vi "CommunicationTool.vi"(0 "VISA资源名称":refnum<visa-resource-name>="COM1", 1 "SN":string, 2 "ModelNumber":string, 5 "通信协议名称":string, 7 "Slot":T1, 9 "DelayTime":u32=1000, 11 "error in":errorcluster, 12 "Debug":bool) -> (3 "字符串数值":bool=TRUE, 4 "响应":string="ÿÿÿÿÿÿÿÿÿÿÿÿÿÿÿÿÿÿÿÿÿÿÿÿÿÿÿ", 6 "反馈结果":bool, 10 "CMD":string, 14 "data":string, 15 "error out":errorcluster)   [LabVIEW 2013]
doc: "本范例根据用户指示，对串口执行读写操作。范例运行时可按下“写入”或“读取”按钮，以及修改“读数”。\n\n设置的串口参数必须匹配连接仪器或设备的参数。本范例中，“读数”参数可指定串口读取的字节数。如端口字节超过指定的字节数，超出部分将不会被读取。如端口字节数少于指定的字节数，将返回超时错误。\n\n本范例可扩展流控制选项以包括XON和XOFF，从而允许用户选择控制字符。同时，用户可启用或禁用中止符。部分设备需要通过终止符确定命令字符串的结束位置。部分设备将发送终止符以说明待读取数据的末端。本范例演示了缓冲区中检测到终止符时，结束“读取”操作或添加终止符至“写入”数据末端的方法。"
uses:
  SystemCode/SysControl/Slot.ctl
  <vilib>/Utility/NIReport.llb/NI_report.lvclass
  SourceCode/CCID info.ctl
  SourceCode/GlobalValue.vi
  <vilib>/Utility/error.llb/Error Cluster From Error Code.vi
  <vilib>/addons/_office/excel.llb/Excel Get Data ([str]).vi
  <vilib>/Utility/file.llb/Write To Spreadsheet File (string).vi
  <vilib>/Utility/file.llb/Read From Spreadsheet File (string).vi
  <vilib>/ErrorRing/Error Ring.xnode
  <vilib>/addons/_office/NI_ReportGenerationToolkit.lvlib
  <vilib>/Utility/NIReport.llb/Excel/NI_Excel.lvclass
panel:
  out "Time(ms)":u32
  out "SerNO":string
  out "硬件版本":string
  out "终端ID":string
  out "CCID":string="PASS"
  out "生产日期":string
  out "字符串":string
  out "x-y":u32
  out "已删除的部分":u8[](array[numeric]) format="%x"
  out "读取缓冲区":string
  out "数据Hex":string[](array[string])
  out "数据ASCII":string[](array[string])
  out "数据类型":string[](array[string])
  in  "命令列表":u16(ring)=17
  out "Write":bool
  out "Read":bool
  out "ConfigPath":string="C:\\Users\\dell\\Desktop\\ExcelReport.vi"
  out "Data":string
  out "DataType":string
  out "命令":string
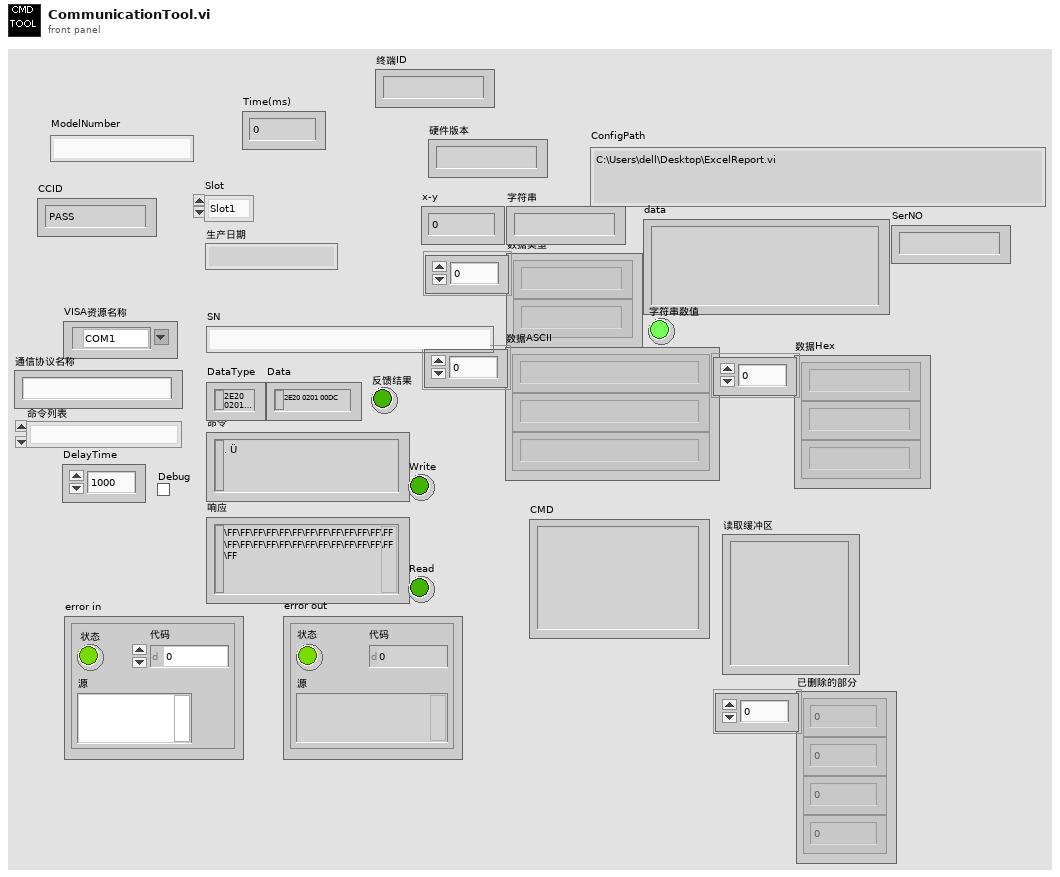
[diagram p1: front panel]
types:
  T1 = typedef "Slot.ctl" = enum16{"Slot1", "Slot2", "Slot3", "Slot4"}
  T2 = enum32{"invalid app kind", "Development System", "Run Time System", "Student Edition", "Embedded LabVIEW", "Evaluation", "Custom"}
  T3 = enum16{"maximized", "minimized", "normal", "no change"}
  T4 = enum16{"Standard Report", "HTML", "Word", "Excel"}
  T5 = typedef "CCID info.ctl" = enum16{"Fw Ver", "HW Ver", "CCID", "WiFiName", "DevID"}
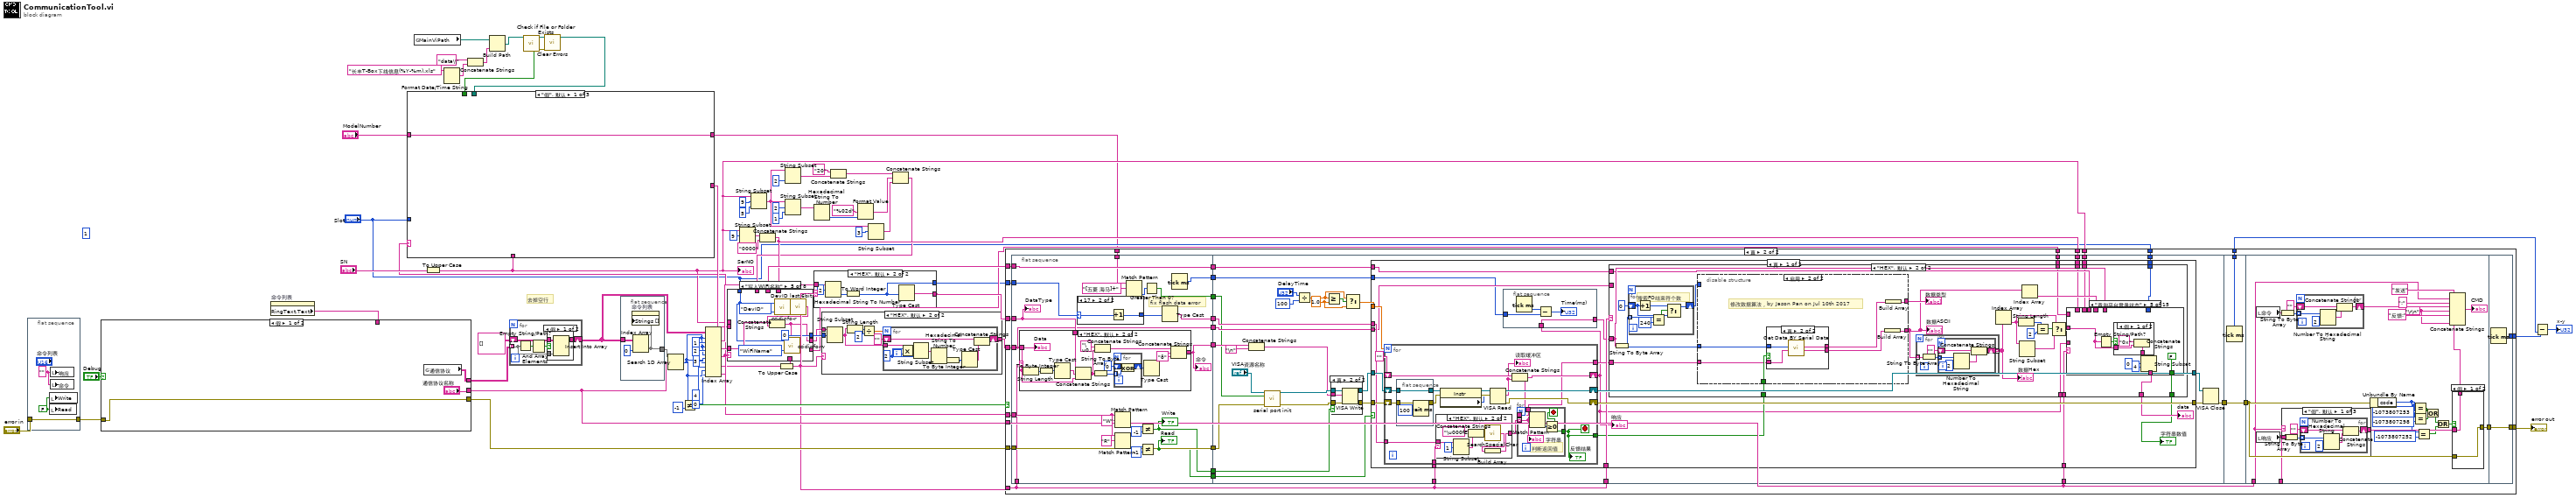
[diagram p0: block diagram]
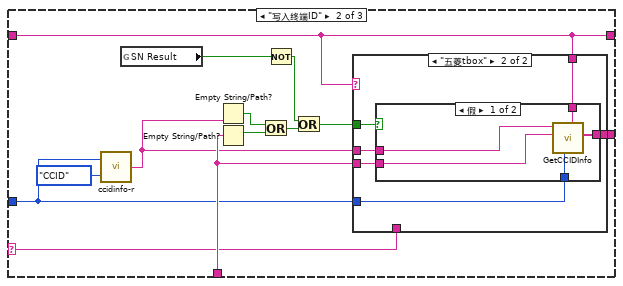
[diagram p2: hidden frame]
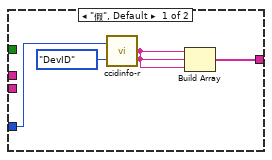
[diagram p3: hidden frame]
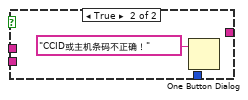
[diagram p4: hidden frame]
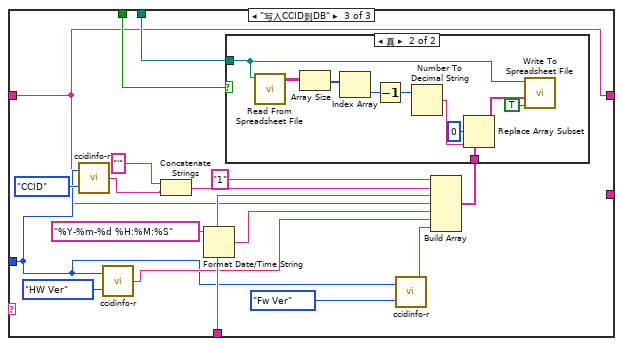
[diagram p5: hidden frame]
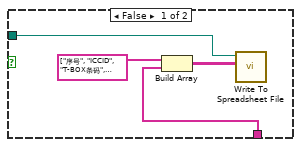
[diagram p6: hidden frame]
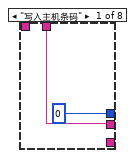
[diagram p7: hidden frame]
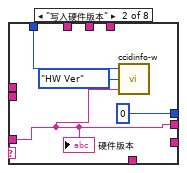
[diagram p8: hidden frame]
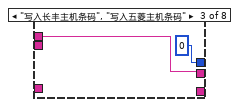
[diagram p9: hidden frame]
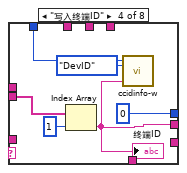
[diagram p10: hidden frame]
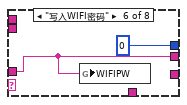
[diagram p11: hidden frame]
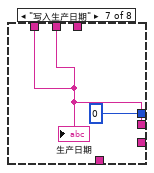
[diagram p12: hidden frame]
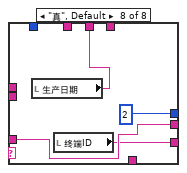
[diagram p13: hidden frame]
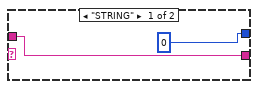
[diagram p14: hidden frame]
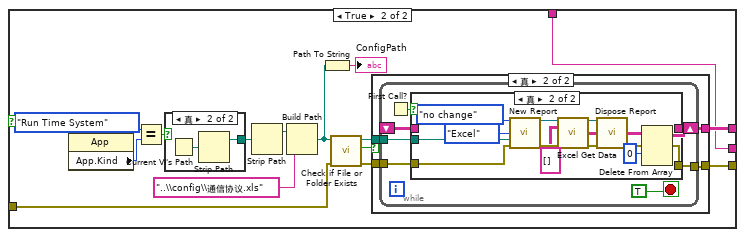
[diagram p17: hidden frame]
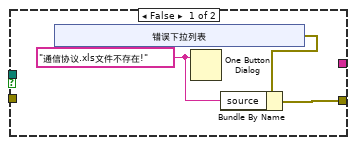
[diagram p18: hidden frame]
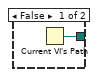
[diagram p20: hidden frame]
diagram:
  (unwired) 1
  # "去掉空行"
  n1 = flat-sequence {
    tunnel: "error in" -> [w71]
    tunnel: [w71] -> w68
    frame #0 {
      w73 = FALSE ("Read")
      w72 = "" ("响应")
      n2 = local write "Write"(w73) -> ()
      n3 = local write "Read"(w73) -> ()
      n4 = local write "响应"(w72) -> ()
      n5 = local write "命令"(w72) -> ()
    }
  }
  n6 = property on="命令列表" class="Ring (严格)"() -> ("RingText.Text"=w67:string)  [unwired: 2 in, 2 out]
  n7 = case shown="假" "Debug" {
    tunnel: [w75 w80] -> w65
    tunnel: w68 -> [w75 w79]
    tunnel: ["通信协议名称" w77] -> w56
    tunnel: [w74 w78] -> w5
    tunnel: w67 -> [_ w77]
    frame False {
      n8 = global read "GlobalValue.vi" "通信协议"() -> (w74:string[][])
    }
    frame True {
      n9 = property class="App"() -> ("App.Kind"=w89:T2)  [unwired: 2 in, 2 out]
      n10 = Equal?(x=T2."Run Time System" ("y"), y=w89) -> (x = y?=w91:bool)
      n11 = case shown="真" w91 {
        tunnel: [w125 w127] -> w90
        frame False {
          n12 = Current VI's Path() -> (path=w125:path)
        }
        frame True {
          n13 = Current VI's Path() -> (path=w126:path)
          n14 = Strip Path(path=w126) -> (stripped path=w127:path)  [unwired: 1 out]
        }
      }
      n15 = Strip Path(path=w90) -> (stripped path=w84:path)  [unwired: 1 out]
      n16 = Build Path(base path=w84, name or relative path="..\\config\\通信协议.xls" ("连接的字符串")) -> (appended path=w86:path)
      n17 = Path To String(path=w86) -> (string=→"ConfigPath":string)
      n18 = call <vilib>:"Check if File or Folder Exists.vi"("error in (no error)"=w79, "path"=w86) -> ("error out"=w81:errorcluster, "file or folder exists?"=w83:bool, "dup path"=w82:path)  [unwired: 7 out]
      n19 = case shown="真" w83 {
        tunnel: w82 -> [_ w102]
        tunnel: w81 -> [_ w101]
        tunnel: [w93 w100] -> w80
        tunnel: [_ w99] -> w78
        frame False {
          w94 = "通信协议.xls文件不存在!" ("消息")
          n20 = xnode "错误下拉列表"() -> ("错误输出"=w92:errorcluster)
          n21 = One Button Dialog(message=w94) -> ()  [unwired: 1 in, 1 out]
          n22 = Bundle By Name(cluster=w92, "source"=w94) -> (w93:errorcluster)
        }
        frame True {
          n23 = while {
            tunnel: w102 -> [w108]
            tunnel: [w107] -> w100
            tunnel: w101 -> [w106]
            shift-right: [w109] -> w99
            shift-left: _ -> [w104]
            stop <- TRUE stop-if-true
            n24 = First Call?() -> (First Call?: T/F=w103:bool)
            n25 = case shown="真" w103 {
              tunnel: [w111 w115] -> w109
              tunnel: w108 -> [_ w114]
              tunnel: [w110 w113] -> w107
              tunnel: w106 -> [w110 w112]
              tunnel: w104 -> [w111 _]
              frame False {
              }
              frame True {
                n26 = call <vilib>:"New Report.vi"("window state (normal)"=T3."no change", "report type"=T4."Excel", "template (empty)"=w114, "error in (no error)"=w112) -> ("report out"=w120:refnum<class "NI_report.lvclass">, "error out"=w121:errorcluster)  [unwired: 2 in, 8 out]
                n27 = call-poly <vilib>:"Excel Get Data.vi"("report in"=w120, "data type"=string[][] [], "error in (no error)"=w121) -> ("report out"=w117:refnum<class "NI_report.lvclass">, "data"=w122:string[][], "error out"=w116:errorcluster)  [unwired: 10 in]
                n28 = call-dynamic "Dispose Report.vi"("report in"=w117, "error in (no error)"=w116) -> ("error out"=w113:errorcluster)  [unwired: 3 in, 10 out]
                n29 = Delete From Array(array=w122, index (row)=0 ("索引 (行)")) -> (array with subset deleted=w115:string[][])  [unwired: 2 in, 1 out]
              }
            }
          }
        }
      }
    }
  }
  n30 = global read "GlobalValue.vi" "MainViPath"() -> (w11:path)
  n31 = To Upper Case(1:"SN") -> (0:w15:string)
  "SerNO" <- w15
  n32 = Format Date/Time String(time format string (%c)="长丰T-Box下线信息(%Y-%m).xls" ("时间格式字符串(%c)")) -> (date/time string=w13:string)  [unwired: 2 in]
  n33 = Concatenate Strings("data\\" ("字符串"), w13) -> (w10:string)
  n34 = Build Path(base path=w11, name or relative path=w10) -> (appended path=w9:path)
  n35 = for {
    tunnel: w5 -> [w128] mode=indexing
    shift-right: [w131] -> w49
    shift-left: string[][] [] -> [w132]
    n36 = Empty String/Path?(string/path=w128) -> (empty?=w130:bool[])
    n37 = And Array Elements(Boolean array=w130) -> (logical AND=w129:bool)
    n38 = case shown="假" w129 {
      tunnel: w132 -> [w135 w136]
      tunnel: [w134 w136] -> w131
      tunnel: w128 -> [w133 _]
      frame False {
        n39 = Insert Into Array(array=w135, new element=w133) -> (w134:string[][])  [unwired: 2 in]
      }
      frame True {
      }
    }
  }
  n40 = call <vilib>:"Check if File or Folder Exists.vi"("path"=w9) -> ("error out"=w8:errorcluster, "file or folder exists?"=w6:bool, "dup path"=w7:path)  [unwired: 8 in]
  n41 = call <vilib>:"Clear Errors.vi"("error in (no error)"=w8) -> ()  [unwired: 6 in, 1 out]
  n42 = flat-sequence {
    tunnel: [w138] -> w55
    tunnel: w49 -> [w137]
    frame #0 {
      n43 = Index Array(array=w137, index (col)=0 ("禁用的索引 (列)")) -> (element=w138:string[])  [unwired: 1 in]
      n44 = property on="命令列表" class="Ring (严格)"("Strings []"=w138) -> ()  [unwired: 2 in, 2 out]
    }
  }
  n45 = Search 1D Array(1D array=w55, element=w56) -> (index of element=w46:i32)  [unwired: 1 in]
  n46 = Not Equal?(x=w46, y=-1) -> (x != y?=w60:bool)
  n47 = Index Array(array=w49, index (row) #1=w46, index (col) #1=1 ("索引 (列)"), index (row) #2=w46, index (col) #2=2 ("索引 (列)"), index (row) #3=w46, index (col) #3=3 ("索引 (列)"), index (row) #4=w46, index (col) #4=4 ("禁用的索引 (列)"), index (row) #5=w46, index (col) #5=0 ("禁用的索引 (列)")) -> (element #1=w59:string, element #2=w44:string, element #3=w51:string, element #4=w53:string, element #5=w17:string)
  n48 = case shown="\"假\", 默认" w17 {
    selector: w17 -> [_ w142 _]
    tunnel: [_ w153 _] -> w20
    tunnel: "ModelNumber" -> [w140 w141 w170]
    tunnel: w15 -> [_ w146 w185]
    tunnel: w7 -> [_ _ w181]
    tunnel: w6 -> [_ _ w180]
    tunnel: "Slot" -> [_ w145 w172]
    tunnel: [w140 w141 w170] -> w2
    frame "假", Default {
    }
    frame "写入终端ID" {
      n49 = call "ccidinfo-r.vi"("Data Type"=CCID_info."CCID", "Slot"=w145) -> ("Data"=w143:string)
      n50 = global read "GlobalValue.vi" "SN Result"() -> (w152:bool)
      n51 = Empty String/Path?(string/path=w143) -> (empty?=w151:bool)
      n52 = Empty String/Path?(string/path=w146) -> (empty?=w150:bool)
      n53 = Or(x=w151, y=w150) -> (x .or. y?=w148:bool)
      n54 = Not(x=w152) -> (.not. x?=w149:bool)
      n55 = Or(x=w149, y=w148) -> (x .or. y?=w147:bool)
      n56 = case shown="\"五菱tbox\"" w141 {
        tunnel: [w157 w163] -> w153
        tunnel: w147 -> [_ w162]
        tunnel: w141 -> [_ w161]
        tunnel: w146 -> [_ w160]
        tunnel: w145 -> [w155 w159]
        tunnel: w143 -> [_ w158]
        tunnel: w142 -> [_ _]
        frame "假", Default {
          n57 = call "ccidinfo-r.vi"("Data Type"=CCID_info."DevID", "Slot"=w155) -> ("Data"=w154:string)
          n58 = Build Array(w154, w154, w154) -> (w157:string[])
        }
        frame "五菱tbox" {
          n59 = case shown="假" w162 {
            tunnel: [w168 _] -> w163
            tunnel: w158 -> [w167 _]
            tunnel: w160 -> [w166 _]
            tunnel: w161 -> [w165 _]
            tunnel: w159 -> [w164 _]
            frame False {
              n60 = call "GetCCIDInfo.vi"("table name"=w165, "Slot"=w164, "SerNO"=w166, "CCID"=w167) -> ("CCID信息"=w168:string[])  [unwired: 7 in]
            }
            frame True {
              n61 = One Button Dialog(message="CCID或主机条码不正确！" ("消息")) -> ()  [unwired: 1 in, 1 out]
            }
          }
        }
      }
    }
    frame "写入CCID到DB" {
      n62 = call "ccidinfo-r.vi"("Data Type"=CCID_info."CCID", "Slot"=w172) -> ("Data"=w176:string)
      n63 = call "ccidinfo-r.vi"("Data Type"=CCID_info."HW Ver", "Slot"=w172) -> ("Data"=w174:string)
      n64 = Concatenate Strings("'", w176) -> (w178:string)
      n65 = Format Date/Time String(time format string (%c)="%Y-%m-%d %H:%M:%S" ("时间格式字符串(%c)")) -> (date/time string=w183:string)  [unwired: 2 in]
      n66 = call "ccidinfo-r.vi"("Data Type"=CCID_info."Fw Ver", "Slot"=w172) -> ("Data"=w171:string)
      n67 = Build Array("1", w178, w185, w170, w183, w174, w171) -> (w182:string[])
      n68 = case shown="真" w180 {
        tunnel: w181 -> [w190 w191]
        tunnel: w182 -> [w189 w195]
        frame False {
          n69 = Build Array(string[] ["序号", "ICCID", "T-BOX条码", "设备型号", "生产日期", "硬件版本", "软件版本"], w189) -> (w188:string[][])
          n70 = call-poly <vilib>:"Write To Spreadsheet File.vi"("2D data"=w188, "file path (dialog if empty)"=w190) -> ()  [unwired: 6 in, 1 out]
        }
        frame True {
          n71 = call-poly <vilib>:"Read From Spreadsheet File.vi"("file path (dialog if empty)"=w191) -> ("all rows"=w200:string[][])  [unwired: 6 in, 4 out]
          n72 = Array Size(array=w200) -> (size(s)=w199:i32[])
          n73 = Index Array(array=w199) -> (element=w198:i32)  [unwired: 1 in]
          n74 = Decrement(x=w198) -> (x-1=w197:i32)
          n75 = Number To Decimal String(number=w197) -> (decimal integer string=w193:string)  [unwired: 1 in]
          n76 = Replace Array Subset(array=w195, new element=w193, index=0 ("索引")) -> (w192:string[])
          n77 = call-poly <vilib>:"Write To Spreadsheet File.vi"("append to file? (new file:F)"=TRUE, "1D data"=w192, "file path (dialog if empty)"=w191) -> ()  [unwired: 5 in, 1 out]
        }
      }
    }
  }
  n78 = String Subset(string=w15, offset (0)=9 ("偏移量(0)")) -> (substring=w39:string)  [unwired: 1 in]
  n79 = String Subset(string=w15, offset (0)=9 ("偏移量(0)"), length (rest)=5 ("长度（剩余）")) -> (substring=w27:string)
  n80 = Concatenate Strings(w39, "0000" ("字符串")) -> (w37:string)
  n81 = To Upper Case(1:w51) -> (0:w3:string)
  n82 = String Subset(string=w27, length (rest)=2 ("长度（剩余）")) -> (substring=w34:string)  [unwired: 1 in]
  n83 = String Subset(string=w27, offset (0)=2 ("偏移量(0)"), length (rest)=1 ("长度（剩余）")) -> (substring=w29:string)
  n84 = Hexadecimal String To Number(string=w29) -> (number=w24:u32)  [unwired: 2 in, 1 out]
  n85 = case shown="\"HEX\", 默认" w3 {
    tunnel: w59 -> [w202 w205]
    tunnel: [w202 w204] -> w58
    tunnel: [i16 0 w203] -> w1
    frame "STRING" {
    }
    frame "HEX", Default {
      n86 = Hexadecimal String To Number(string=w205, offset=2 ("偏移量")) -> (number=w207:u32)  [unwired: 1 in, 1 out]
      n87 = To Word Integer(number=w207) -> (16bit integer=w203:i16)
      n88 = Type Cast(x=w203) -> (*(type *) &x=w204:string)  [unwired: 1 in]
    }
  }
  n89 = Concatenate Strings("20" ("字符串"), w34) -> (w26:string)
  n90 = Format Value(format string="%02d" ("格式字符串"), value (0)=w24) -> (output string=w22:string)  [unwired: 1 in]
  n91 = String Subset(string=w27, offset (0)=3 ("偏移量(0)")) -> (substring=w25:string)  [unwired: 1 in]
  n92 = Concatenate Strings(w26, w22, w25) -> (w21:string)
  n93 = case shown="\"写入WIFI名称\"" w17 {
    tunnel: w44 -> [_ w210 _ _ w228 w230 _ w237]
    tunnel: [w208 w210 w214 w216 w224 w230 w232 w237] -> w19
    tunnel: [0 ("偏移量(0)") 0 ("偏移量(0)") 0 ("偏移量(0)") 0 ("偏移量(0)") 0 ("偏移量(0)") 0 ("偏移量(0)") 0 ("偏移量(0)") 2 ("偏移量(0)")] -> w43
    tunnel: [_ _ _ _ _ _ w232 w235] -> w41
    tunnel: w37 -> [w208 _ _ _ _ _ _ _]
    tunnel: w21 -> [_ _ _ _ _ _ w232 _]
    tunnel: w15 -> [_ _ w214 _ _ _ _ _]
    tunnel: w20 -> [_ _ _ w220 _ _ _ _]
    tunnel: [_ _ _ _ _ _ _ w234] -> w18
    tunnel: "Slot" -> [_ w212 _ w217 w225 _ _ _]
    tunnel: w3 -> [_ _ _ _ _ _ _ _]
    frame "写入主机条码" {
    }
    frame "写入硬件版本" {
      n94 = call "ccidinfo-w.vi"("Data"=w210, "Data Type"=CCID_info."HW Ver", "Slot"=w212) -> ()  [unwired: 1 in]
      "硬件版本" <- w210
    }
    frame "写入长丰主机条码", "写入五菱主机条码" {
    }
    frame "写入终端ID" {
      n95 = Index Array(array=w220, index=1 ("索引")) -> (element=w216:string)
      "终端ID" <- w216
      n96 = call "ccidinfo-w.vi"("Data"=w216, "Data Type"=CCID_info."DevID", "Slot"=w217) -> ()  [unwired: 1 in]
    }
    frame "写入WIFI名称" {
      n97 = call "ccidinfo-r.vi"("Data Type"=CCID_info."DevID", "Slot"=w225) -> ("Data"=w223:string)
      n98 = call "DevID last 6bit.vi"("Devid"=w223) -> ("结果字符串"=w222:string)  [unwired: 4 in]
      n99 = Concatenate Strings(w228, w222) -> (w224:string)
      n100 = call "ccidinfo-w.vi"("Data"=w224, "Data Type"=CCID_info."WiFiName", "Slot"=w225) -> ()  [unwired: 1 in]
    }
    frame "写入WIFI密码" {
      n101 = global write "GlobalValue.vi" "WIFIPW"(w230) -> ()
    }
    frame "写入生产日期" {
      "生产日期" <- w232
    }
    frame "真", Default {
      n102 = local read "生产日期"() -> (w235:string)
      n103 = local read "终端ID"() -> (w234:string)
    }
  }
  n104 = case shown="\"HEX\", 默认" w3 {
    tunnel: [w238 w243] -> w57
    tunnel: w19 -> [w238 w242]
    tunnel: w43 -> [_ w239]
    frame "ASCII" {
    }
    frame "HEX", Default {
      n105 = String Subset(string=w242, offset (0)=w239) -> (substring=w241:string)  [unwired: 1 in]
      n106 = String Length(string=w241) -> (length=w245:i32)
      n107 = Divide(x=w245, y=2) -> (x/y=w240:dbl)
      n108 = for {
        N: w240 -> [_]
        tunnel: w241 -> [w251]
        shift-right: [w253] -> w243
        shift-left: "" -> [w252]
        i -> [w249]
        w247 = 2 ("x")
        n109 = Multiply(x=w247, y=w249) -> (x*y=w248:i32)
        n110 = String Subset(string=w251, offset (0)=w248, length (rest)=w247) -> (substring=w250:string)
        n111 = Hexadecimal String To Number(string=w250) -> (number=w256:u32)  [unwired: 2 in, 1 out]
        n112 = To Byte Integer(number=w256) -> (8bit integer=w255:i8)
        n113 = Type Cast(x=w255) -> (*(type *) &x=w254:string)  [unwired: 1 in]
        n114 = Concatenate Strings(w252, w254) -> (w253:string)
      }
    }
  }
  n115 = case shown="真" w60 {
    tunnel: w56 -> [w261 w278]
    tunnel: w58 -> [_ w289]
    tunnel: w57 -> [_ w288]
    tunnel: w65 -> [_ w287]
    tunnel: [w257 w285] -> w70
    tunnel: w53 -> [_ w284]
    tunnel: w3 -> [_ w279]
    tunnel: [_ w274] -> w66
    tunnel: [_ w273] -> w48
    tunnel: w41 -> [_ w272]
    tunnel: w37 -> [_ w270]
    tunnel: w15 -> [_ w269]
    tunnel: w18 -> [_ w268]
    tunnel: "Slot" -> [_ w265]
    tunnel: w2 -> [_ w264]
    tunnel: w1 -> [_ w262]
    frame False {
      (unwired) "FF" ("响应")
      n116 = Concatenate Strings(w261, "名称不存在" ("消息")) -> (w258:string)
      n117 = One Button Dialog(message=w258) -> ()  [unwired: 1 in, 1 out]
      n118 = Bundle By Name(cluster=errorcluster {"status"=TRUE, "code"=5000, "source"=""} ("error in 1 (no error)"), "source"=w258) -> (w257:errorcluster)
    }
    frame True {
      n119 = flat-sequence {
        tunnel: w289 -> [w301]
        tunnel: w288 -> [w298]
        tunnel: w287 -> [w312]
        tunnel: [w312] -> w286
        tunnel: w284 -> [w311]
        tunnel: [w304] -> w283
        tunnel: [w303] -> w282
        tunnel: [w302] -> w281
        tunnel: [w290] -> w280
        tunnel: w279 -> [w300]
        tunnel: w272 -> [w299]
        tunnel: [w299] -> w271
        tunnel: [w298] -> w267
        tunnel: [w297] -> w266
        tunnel: w264 -> [w296]
        tunnel: [w293] -> w263
        tunnel: w262 -> [w292]
        tunnel: w286 -> [w365]
        tunnel: w283 -> [w360]
        tunnel: w282 -> [w363]
        tunnel: [w364] -> w277
        tunnel: w281 -> [w339]
        tunnel: w280 -> [w359]
        tunnel: w279 -> [w350]
        tunnel: w279 -> [w349]
        tunnel: w278 -> [w348]
        tunnel: w271 -> [w347]
        tunnel: w270 -> [w346]
        tunnel: w269 -> [w345]
        tunnel: w268 -> [w344]
        tunnel: w267 -> [w343]
        tunnel: w266 -> [w342]
        tunnel: w265 -> [w341]
        tunnel: w263 -> [w336]
        tunnel: w277 -> [w714]
        tunnel: [w714] -> w276
        tunnel: [w713] -> w273
        tunnel: w276 -> [w727]
        tunnel: w278 -> [w715]
        tunnel: [w716] -> _
        tunnel: [w728] -> w275
        tunnel: [w760] -> w285
        tunnel: w275 -> [w760]
        tunnel: [w759] -> w274
        frame #0 {
          # "fix flash data error"
          n120 = case shown="\"HEX\", 默认" w300 {
            tunnel: w298 -> [w317 w329]
            tunnel: [w316 w323] -> w302
            tunnel: w301 -> [w318 w322]
            frame "STRING" {
              n121 = Concatenate Strings(w318, w317) -> (w316:string)
            }
            frame "HEX", Default {
              n122 = String Length(string=w329) -> (length=w320:i32)
              n123 = To Byte Integer(number=w320) -> (8bit integer=w321:i8)
              n124 = Type Cast(x=w321) -> (*(type *) &x=w319:string)  [unwired: 1 in]
              n125 = Concatenate Strings(w322, w319, w329) -> (w332:string)
              n126 = String To Byte Array(string=w332) -> (unsigned byte array=w328:u8[])
              n127 = Concatenate Strings("\u000f" ("HeadCode"), w332) -> (w325:string)
              n128 = for {
                tunnel: w328 -> [w335] mode=indexing
                shift-right: [w333] -> w326
                shift-left: u8 0 ("y") -> [w334]
                n129 = Exclusive Or(1:w335, 2:w334) -> (0:w333:u8)
              }
              n130 = Type Cast(x=w326) -> (*(type *) &x=w330:string)  [unwired: 1 in]
              n131 = Concatenate Strings(w325, w330, "ð" ("字符串")) -> (w323:string)
              "Data" <- w329
            }
          }
          "命令" <- w302
          n132 = case shown="17" w292 {
            selector: w292 -> [w313 w315]
            tunnel: [w313 w314] -> w291
            frame 0, Default {
            }
            frame 17 {
              n133 = Increment(x=w315) -> (x+1=w314:i16)
            }
          }
          n134 = Match Pattern(string=w311, regular expression="W" ("正则表达式")) -> (offset past match=w305:i32)  [unwired: 1 in, 3 out]
          n135 = Match Pattern(string=w311, regular expression="R" ("正则表达式")) -> (offset past match=w306:i32)  [unwired: 1 in, 3 out]
          n136 = Match Pattern(string=w296, regular expression="[五菱 海马]+" ("正则表达式")) -> (offset past match=w294:i32)  [unwired: 1 in, 3 out]
          n137 = Not Equal?(x=w305, y=-1) -> (x != y?=w304:bool)
          "Write" <- w304
          n138 = Not Equal?(x=w306, y=-1) -> (x != y?=w303:bool)
          "Read" <- w303
          n139 = Greater Than 0?(x=w294) -> (x > 0?=w293:bool)
          n140 = Type Cast(x=w291) -> (*(type *) &x=w290:string)  [unwired: 1 in]
          n141 = Tick Count (ms)() -> (millisecond timer value=w297:u32)
          "DataType" <- w301
        }
        frame #1 {
          w356 = 1.0 ("y")
          n142 = Concatenate Strings(w339, "\n") -> (w337:string)
          n143 = call "serial port init.vi"("错误输入（无错误）"=w365, "海马(1)"=w336, "VISA引用句柄输入"="VISA资源名称") -> ("错误输出"=w361:errorcluster, "VISA引用句柄输出"=w362:refnum<visa-resource-name>)  [unwired: 7 in]
          n144 = Divide(x="DelayTime", y=u32 100) -> (x/y=w355:dbl)
          n145 = Greater Or Equal?(x=w355, y=w356) -> (x >= y?=w354:bool)
          n146 = case shown="真" w360 {
            tunnel: w362 -> [w369 w374]
            tunnel: [w369 w373] -> w358
            tunnel: [w368 w372] -> w357
            tunnel: w361 -> [w368 w371]
            tunnel: w337 -> [_ w370]
            frame False {
            }
            frame True {
              n147 = VISA Write(VISA resource name=w374, write buffer=w370, error in (no error)=w371) -> (VISA resource name out=w373:refnum<visa-resource-name>, error out=w372:errorcluster)  [unwired: 1 out]
            }
          }
          n148 = Select(t=w355, s=w354, f=w356) -> (s? t:f=w351:dbl)
          n149 = case shown="真" w363 {
            tunnel: [w396 w712] -> w366
            tunnel: w358 -> [w395 w712]
            tunnel: [w397 w711] -> w367
            tunnel: w357 -> [w394 w711]
            tunnel: w359 -> [w392 _]
            tunnel: w351 -> [w391 _]
            tunnel: w350 -> [w390 _]
            tunnel: w349 -> [w389 _]
            tunnel: w348 -> [w387 _]
            tunnel: w347 -> [w384 _]
            tunnel: w346 -> [w383 _]
            tunnel: w345 -> [w382 _]
            tunnel: w344 -> [w381 _]
            tunnel: w343 -> [w380 _]
            tunnel: w342 -> [w379 _]
            tunnel: w341 -> [w377 _]
            frame True {
              n150 = for {
                N: w391 -> [_]
                shift-right: [w695] -> w397
                shift-left: w394 -> [w685]
                shift-right: [w683] -> w375
                shift-left: "" ("read buffer") -> [w690]
                shift-right: [w694] -> w396
                shift-left: w395 -> [w684]
                tunnel: w392 -> [w680]
                tunnel: w390 -> [w682]
                tunnel: [w681] -> w388
                tunnel: [w679] -> w376
                stop <- w681 stop-if-true
                n151 = flat-sequence {
                  tunnel: w685 -> [w710]
                  tunnel: [w710] -> w686
                  tunnel: [w709] -> w687
                  tunnel: w684 -> [w709]
                  frame #0 {
                    n152 = Wait (ms)(milliseconds to wait=u32 100 ("等待时间（毫秒）")) -> ()  [unwired: 1 out]
                  }
                }
                n153 = case shown="\"HEX\", 默认" w682 {
                  tunnel: [string[] ["0x0000000", "create auto test task"] w701] -> w689
                  tunnel: w680 -> [_ w707]
                  frame "STRING" {
                  }
                  frame "HEX", Default {
                    n154 = String Subset(string=w707, offset (0)=1 ("偏移量(0)")) -> (substring=w704:string)  [unwired: 1 in]
                    n155 = Concatenate Strings("\u000f€" ("正则表达式"), w704) -> (w703:string)
                    n156 = call "SearchSpecialChar.vi"("正则表达式"=w703) -> ("字符串"=w702:string)
                    n157 = Build Array(w702) -> (w701:string[])
                  }
                }
                n158 = property class="Instr"(reference=w687, error in=w686) -> (reference out=w693:refnum<visa-resource-name>, error out=w692:errorcluster, "Serial Settings:Number of Bytes at Serial Port"=w691:u32)
                n159 = VISA Read(VISA resource name=w693, byte count=w691, error in (no error)=w692) -> (VISA resource name out=w694:refnum<visa-resource-name>, read buffer=w688:string, error out=w695:errorcluster)  [unwired: 1 out]
                "读取缓冲区" <- w688
                n160 = Concatenate Strings(w690, w688) -> (w683:string)
                n161 = for {
                  tunnel: w689 -> [w696] mode=indexing
                  tunnel: w683 -> [w698]
                  tunnel: [w697] -> w681
                  tunnel: [w696] -> w679
                  stop <- w697 stop-if-true
                  # "判断返回值"
                  n162 = Match Pattern(string=w698, regular expression=w696) -> (offset past match=w699:i32)  [unwired: 1 in, 3 out]
                  n163 = Greater Or Equal To 0?(x=w699) -> (x >= 0?=w697:bool)
                  "字符串" <- w696
                }
                "反馈结果" <- w681
              }
              "响应" <- w375
              n164 = flat-sequence {
                tunnel: w379 -> [w399]
                tunnel: w375 -> [w398]
                tunnel: [w398] -> w378
                frame #0 {
                  n165 = Tick Count (ms)() -> (millisecond timer value=w400:u32)
                  n166 = Subtract(x=w400, y=w399) -> (x-y=→"Time(ms)":u32)
                }
              }
              n167 = case shown="\"HEX\", 默认" w389 {
                tunnel: w378 -> [w408 w479]
                tunnel: w388 -> [w405 w471]
                tunnel: w387 -> [w409 w487]
                tunnel: [w407 w486] -> w386
                tunnel: [w406 w485] -> w385
                tunnel: w384 -> [_ w476]
                tunnel: w383 -> [_ w475]
                tunnel: w382 -> [w403 w474]
                tunnel: w381 -> [_ w473]
                tunnel: w380 -> [w404 _]
                tunnel: w377 -> [w402 w472]
                tunnel: w376 -> [_ w470]
                tunnel: w375 -> [_ w469]
                frame "STRING" {
                  n168 = case shown="\"查询版本(1701)\"" w409 {
                    tunnel: [w410 w419 w442] -> w407
                    tunnel: [FALSE FALSE FALSE] -> w406
                    tunnel: w408 -> [_ w426 w450]
                    tunnel: w405 -> [w411 _ _]
                    tunnel: w404 -> [_ w421 w444]
                    tunnel: w403 -> [_ _ _]
                    tunnel: w402 -> [_ w417 w440]
                    frame "真", Default {
                      n169 = Select(t="OK", s=w411, f="") -> (s? t:f=w410:string)
                    }
                    frame "查询版本", "查询版本(长丰)" {
                      # "查询版本指令--修改兼容海马,五菱,长丰  --- by Jason Pan on Jan 20th 2017"
                      n170 = Concatenate Strings(w421, "\n" ("字符串")) -> (w420:string)
                      n171 = Match Pattern(string=w426, regular expression=w420) -> (after substring=w425:string)  [unwired: 1 in, 3 out]
                      n172 = for {
                        tunnel: w425 -> [w439]
                        tunnel: [w438] -> w423
                        tunnel: string[] ["\r\n\t1, 0x00000001\r\ncmd>", "\r\n\t0, 0x00000000\r\ncmd>", "\n\t0, 0x00000000", "\r\ncmd>"] -> [w435] mode=indexing
                        tunnel: [w434] -> w424
                        i -> [w434]
                        stop <- w436 stop-if-true
                        n173 = Match Pattern(string=w439, regular expression=w435) -> (before substring=w438:string, offset past match=w437:i32)  [unwired: 1 in, 2 out]
                        n174 = Greater Or Equal To 0?(x=w437) -> (x >= 0?=w436:bool)
                      }
                      n175 = case shown="0, 默认" w424 {
                        tunnel: [w428 w429] -> w422
                        tunnel: w423 -> [w428 w433]
                        frame 0, Default {
                          # "海马/长丰tbox"
                        }
                        frame 3 {
                          # "五菱tbox"
                          n176 = Match Pattern(string=w433, regular expression="app start,version:" ("正则表达式")) -> (after substring=w431:string)  [unwired: 1 in, 3 out]
                          n177 = Match Pattern(string=w431, regular expression="\r\n" ("正则表达式")) -> (before substring=w429:string)  [unwired: 1 in, 3 out]
                        }
                      }
                      n178 = call <vilib>:"Trim Whitespace.vi"("string"=w422) -> ("trimmed string"=w419:string)  [unwired: 1 in]
                      n179 = call "ccidinfo-w.vi"("Data"=w419, "Data Type"=CCID_info."Fw Ver", "Slot"=w417) -> ()  [unwired: 1 in]
                    }
                    frame "查询版本(1701)" {
                      # "查询版本指令--修改兼容海马,五菱,长丰  --- by Jason Pan on Jan 20th 2017"
                      n180 = Concatenate Strings(w444) -> (w443:string)
                      n181 = Match Pattern(string=w450, regular expression=w443) -> (after substring=w449:string)  [unwired: 1 in, 3 out]
                      n182 = for {
                        tunnel: w449 -> [w468]
                        tunnel: [w467] -> w446
                        tunnel: string[] ["\r\nAES", "\nAES"] -> [w464] mode=indexing
                        tunnel: [w463] -> w447
                        i -> [w463]
                        stop <- w465 stop-if-true
                        n183 = Match Pattern(string=w468, regular expression=w464) -> (before substring=w467:string, offset past match=w466:i32)  [unwired: 1 in, 2 out]
                        n184 = Greater Or Equal To 0?(x=w466) -> (x >= 0?=w465:bool)
                      }
                      n185 = case shown="0" w447 {
                        tunnel: [w452 w453 w458] -> w445
                        tunnel: w446 -> [w452 w457 w462]
                        frame -1, Default {
                          # "海马/长丰tbox"
                        }
                        frame 0 {
                          # "tbox/1701"
                          n186 = Match Pattern(string=w457, regular expression="app start,version:" ("正则表达式")) -> (after substring=w455:string)  [unwired: 1 in, 3 out]
                          n187 = Match Pattern(string=w455, regular expression="\r\n" ("正则表达式")) -> (before substring=w453:string)  [unwired: 1 in, 3 out]
                        }
                        frame 1 {
                          # "1701"
                          n188 = Match Pattern(string=w462, regular expression="app start,version:" ("正则表达式")) -> (after substring=w460:string)  [unwired: 1 in, 3 out]
                          n189 = Match Pattern(string=w460, regular expression="\n" ("正则表达式")) -> (before substring=w458:string)  [unwired: 1 in, 3 out]
                        }
                      }
                      n190 = call <vilib>:"Trim Whitespace.vi"("string"=w445) -> ("trimmed string"=w442:string)  [unwired: 1 in]
                      n191 = call "ccidinfo-w.vi"("Data"=w442, "Data Type"=CCID_info."Fw Ver", "Slot"=w440) -> ()  [unwired: 1 in]
                    }
                  }
                }
                frame "HEX", Default {
                  n192 = String To Byte Array(string=w479) -> (unsigned byte array=w484:u8[])
                  n193 = for {
                    tunnel: w484 -> [w553] mode=indexing
                    shift-right: [w549] -> w482
                    shift-left: 0 ("y") -> [w548]
                    # "搜索FO结束符个数"
                    n194 = Increment(x=w548) -> (x+1=w550:i32)
                    n195 = Equal?(x=w553, y=u8 240) -> (x = y?=w551:bool)
                    n196 = Select(t=w550, s=w551, f=w548) -> (s? t:f=w549:i32)
                  }
                  n197 = disable-structure shown="启用" {
                    disable-tunnel: w484 -> [w497 w533]
                    disable-tunnel: w482 -> [w496 _]
                    disable-tunnel: [w495 w531] -> w481
                    disable-tunnel: [w494 w530] -> w478
                    disable-tunnel: w471 -> [_ w528]
                    disable-tunnel: w470 -> [_ w527]
                    frame Disabled {
                      n198 = for {
                        N: w496 -> [_]
                        shift-right: [w520] -> _
                        shift-left: w497 -> [w521]
                        tunnel: [w504] -> w494 mode=indexing
                        tunnel: [w500] -> w495 mode=indexing
                        stop <- w518 stop-if-true
                        # "删除数据类型和两位长度，删除校验码"
                        # "下一个OF和FO的消息处理"
                        # "获取OF和FO之间的数据"
                        n199 = Search 1D Array(1D array=w521, element=u8 15 ("元素")) -> (index of element=w523:i32)  [unwired: 1 in]
                        n200 = Search 1D Array(1D array=w521, element=u8 240 ("元素")) -> (index of element=w516:i32)  [unwired: 1 in]
                        n201 = Increment(x=w523) -> (x+1=w522:i32)
                        n202 = Equal?(x=w516, y=-1) -> (x = y?=w518:bool)
                        n203 = Subtract(x=w516, y=w522) -> (x-y=w524:i32)
                        n204 = Increment(x=w516) -> (x+1=w517:i32)
                        n205 = Array Subset(array=w521, index=w522, length=w524) -> (w513:u8[])
                        n206 = Array Subset(array=w521, index=w517) -> (w520:u8[])  [unwired: 1 in]
                        n207 = Index Array(array=w513) -> (element #1=w514:u8, element #2=w503:u8)  [unwired: 2 in]
                        n208 = Delete From Array(array=w513, length=3 ("长度"), index=0 ("索引")) -> (deleted portion=→"已删除的部分":u8[], array with subset deleted=w510:u8[])
                        n209 = Reverse 1D Array(array=w510) -> (reversed array=w509:u8[])
                        n210 = Number To Hexadecimal String(1:i16 2 ("宽度(-)"), 2:w514) -> (0:w501:string)
                        n211 = Number To Hexadecimal String(1:i16 2 ("宽度(-)"), 2:w503) -> (0:w502:string)
                        n212 = Delete From Array(array=w509, length=1 ("长度"), index=0 ("索引")) -> (array with subset deleted=w506:u8[])  [unwired: 1 out]
                        n213 = Reverse 1D Array(array=w506) -> (reversed array=w505:u8[])
                        n214 = Concatenate Strings(w501, w502) -> (w500:string)
                        n215 = Byte Array To String(unsigned byte array=w505) -> (string=w504:string)
                      }
                    }
                    frame Enabled {
                      # "修改数据算法，by Jason Pan on Jul 10th 2017"
                      n216 = case shown="真" w528 {
                        tunnel: w533 -> [_ w538]
                        tunnel: [w534 w537] -> w532
                        tunnel: [w534 w536] -> w529
                        tunnel: w527 -> [_ w535]
                        frame False {
                          w534 = ""
                        }
                        frame True {
                          n217 = call "Get Data BY Serial Data.vi"("HEAD"=w535, "Data in"=w538) -> ("Data"=w536:string, "Data Type"=w537:string)  [unwired: 8 in]
                        }
                      }
                      n218 = Build Array(w529) -> (w530:string[])
                      n219 = Build Array(w532) -> (w531:string[])
                    }
                  }
                  "数据类型" <- w481
                  "数据ASCII" <- w478
                  n220 = for {
                    tunnel: w478 -> [w542] mode=indexing
                    tunnel: [w539] -> w480 mode=indexing
                    n221 = String To Byte Array(string=w542) -> (unsigned byte array=w540:u8[])
                    n222 = for {
                      tunnel: w540 -> [w547] mode=indexing
                      shift-right: [w545] -> w539
                      shift-left: "" -> [w544]
                      n223 = Number To Hexadecimal String(1:i16 2 ("宽度(-)"), 2:w547) -> (0:w546:string)
                      n224 = Concatenate Strings(w544, w546) -> (w545:string)
                    }
                  }
                  "数据Hex" <- w480
                  n225 = Index Array(array=w480) -> (element=w490:string)  [unwired: 1 in]
                  n226 = String Length(string=w490) -> (length=w493:i32)
                  n227 = String Subset(string=w490) -> (substring=w489:string)  [unwired: 2 in]
                  n228 = Index Array(array=w478) -> (element=w477:string)  [unwired: 1 in]
                  n229 = Equal?(x=w493, y=2) -> (x = y?=w491:bool)
                  n230 = Select(t=w490, s=w491, f=w489) -> (s? t:f=w488:string)
                  n231 = case shown="\"查询平台登录状态\"" w487 {
                    tunnel: w488 -> [w556 w569 w573 w576 w587 _ _ _ _ _ _ _ _ _ _]
                    tunnel: [w555 w565 w571 w577 w584 w593 w596 w604 w617 w625 w635 w643 w654 w664 w674] -> w486
                    tunnel: [TRUE TRUE TRUE FALSE FALSE FALSE TRUE FALSE FALSE FALSE FALSE FALSE FALSE FALSE FALSE] -> w485
                    tunnel: w479 -> [_ _ _ _ _ _ w600 _ _ _ _ _ _ _ _]
                    tunnel: w477 -> [_ _ _ _ _ _ _ w608 w616 w623 w632 w651 w658 w661 w672]
                    tunnel: w476 -> [_ _ _ _ _ _ _ _ _ _ _ _ w653 _ _]
                    tunnel: w475 -> [_ _ _ _ _ _ _ w602 _ _ _ _ _ _ _]
                    tunnel: w474 -> [_ _ _ _ _ _ _ _ _ _ w633 _ _ _ _]
                    tunnel: w473 -> [_ _ _ _ _ _ _ _ _ _ _ _ _ w663 _]
                    tunnel: w472 -> [_ _ _ _ _ _ _ _ w611 _ _ w642 _ _ w670]
                    tunnel: w469 -> [_ _ _ _ _ w594 _ _ _ _ _ _ _ _ _]
                    frame "查询BAT7.2V_DET电压" {
                      n232 = Hexadecimal String To Number(string=w556) -> (number=w559:u32)  [unwired: 2 in, 1 out]
                      n233 = Divide(x=w559, y=u32 1000) -> (x/y=w557:dbl)
                      n234 = Number To Fractional String(number=w557) -> (F-format string=w555:string)  [unwired: 3 in]
                    }
                    frame "查询BAT_DET状态" {
                      n235 = Hexadecimal String To Number(string=w569) -> (number=w567:u32)  [unwired: 2 in, 1 out]
                      n236 = Multiply(x=w567, y=u32 11) -> (x*y=w566:u32)
                      n237 = Divide(x=w566, y=u32 1000) -> (x/y=w562:dbl)
                      n238 = Add(x=w562, y=0.3) -> (x+y=w560:dbl)
                      n239 = Number To Fractional String(number=w560) -> (F-format string=w565:string)  [unwired: 3 in]
                    }
                    frame "加速度传感器返回数据1" {
                      n240 = Hexadecimal String To Number(string=w573) -> (number=w572:u32)  [unwired: 2 in, 1 out]
                      n241 = Number To Decimal String(number=w572) -> (decimal integer string=w571:string)  [unwired: 1 in]
                    }
                    frame "真", Default {
                      n242 = Empty String/Path?(string/path=w576) -> (empty?=w575:bool)
                      n243 = case shown="假" w575 {
                        tunnel: [w579 ""] -> w577
                        tunnel: w576 -> [w578 _]
                        frame False {
                          n244 = Concatenate Strings("0x" ("字符串"), w578) -> (w579:string)
                        }
                        frame True {
                        }
                      }
                    }
                    frame "查询平台登录状态" {
                      n245 = Empty String/Path?(string/path=w587) -> (empty?=w586:bool)
                      n246 = case shown="假" w586 {
                        tunnel: [w590 ""] -> w588
                        tunnel: w587 -> [w589 _]
                        frame False {
                          n247 = Concatenate Strings("0x" ("字符串"), w589) -> (w590:string)
                        }
                        frame True {
                        }
                      }
                      n248 = String Subset(string=w588, offset (0)=0 ("长度（剩余）"), length (rest)=4 ("长度（剩余）")) -> (substring=w584:string)
                    }
                    frame "查询4G固件版本" {
                      n249 = call "VerStringTrim.vi"("读取缓冲区"=w594) -> ("结果"=w593:string)
                    }
                    frame "查询版本" {
                      n250 = Match Pattern(string=w600, regular expression="ver()\r\n" ("正则表达式")) -> (after substring=w598:string)  [unwired: 1 in, 3 out]
                      n251 = Match Pattern(string=w598, regular expression="\r\n\t1, 0x00000001\r\ncmd>" ("正则表达式")) -> (before substring=w596:string)  [unwired: 1 in, 3 out]
                    }
                    frame "读出主机条码" {
                      n252 = To Upper Case(1:w602) -> (0:w603:string)
                      n253 = Equal?(x=w608, y=w603) -> (x = y?=w607:bool)
                      n254 = Select(t="PASS" ("string"), s=w607, f="FAIL") -> (s? t:f=w604:string)
                    }
                    frame "读出WIFI名称" {
                      n255 = call "ccidinfo-r.vi"("Data Type"=CCID_info."WiFiName", "Slot"=w611) -> ("Data"=w610:string)
                      n256 = To Upper Case(1:w610) -> (0:w614:string)
                      n257 = Match Pattern(string=w616, regular expression=w614) -> (match substring=w615:string)  [unwired: 1 in, 3 out]
                      n258 = Equal?(x=w615, y=w614) -> (x = y?=w613:bool)
                      n259 = Select(t="PASS" ("string"), s=w613, f="FAIL") -> (s? t:f=w617:string)
                    }
                    frame "读出WIFI密码" {
                      n260 = global read "GlobalValue.vi" "WIFIPW"() -> (w624:string)
                      n261 = To Upper Case(1:w624) -> (0:w621:string)
                      n262 = Match Pattern(string=w623, regular expression=w621) -> (match substring=w622:string)  [unwired: 1 in, 3 out]
                      n263 = Equal?(x=w622, y=w621) -> (x = y?=w628:bool)
                      n264 = Select(t="PASS" ("string"), s=w628, f="FAIL") -> (s? t:f=w625:string)
                    }
                    frame "读出长丰主机条码", "读出五菱主机条码" {
                      n265 = To Upper Case(1:w633) -> (0:w634:string)
                      n266 = String Subset(string=w632, offset (0)=1 ("偏移量(0)")) -> (substring=w630:string)  [unwired: 1 in]
                      n267 = Equal?(x=w630, y=w634) -> (x = y?=w638:bool)
                      n268 = Select(t="PASS" ("string"), s=w638, f="FAIL") -> (s? t:f=w635:string)
                    }
                    frame "读出CCID" {
                      n269 = String Subset(string=w651, offset (0)=1 ("偏移量(0)")) -> (substring=w649:string)  [unwired: 1 in]
                      n270 = To Upper Case(1:w649) -> (0:w640:string)
                      "CCID" <- w640
                      n271 = String Length(string=w640) -> (length=w646:i32)
                      n272 = Equal?(x=w646, y=20) -> (x = y?=w644:bool)
                      n273 = Select(t="PASS" ("string"), s=w644, f="FAIL") -> (s? t:f=w643:string)
                      n274 = call "ccidinfo-w.vi"("Data"=w640, "Data Type"=CCID_info."CCID", "Slot"=w642) -> ()  [unwired: 1 in]
                    }
                    frame "读出生产日期" {
                      n275 = Equal?(x=w658, y=w653) -> (x = y?=w657:bool)
                      n276 = Select(t="PASS" ("string"), s=w657, f="FAIL") -> (s? t:f=w654:string)
                    }
                    frame "读出终端ID" {
                      n277 = String Subset(string=w661, offset (0)=1 ("偏移量(0)")) -> (substring=w660:string)  [unwired: 1 in]
                      n278 = Equal?(x=w660, y=w663) -> (x = y?=w667:bool)
                      n279 = Select(t="PASS" ("string"), s=w667, f="FAIL") -> (s? t:f=w664:string)
                    }
                    frame "读出硬件版本" {
                      n280 = call "Set HW data.vi"("Slot"=w670) -> ("HW DATA"=w669:string)  [unwired: 4 in]
                      n281 = String Subset(string=w672, offset (0)=1 ("偏移量(0)")) -> (substring=w671:string)  [unwired: 1 in]
                      n282 = Equal?(x=w671, y=w669) -> (x = y?=w677:bool)
                      n283 = Select(t="PASS" ("string"), s=w677, f="FAIL") -> (s? t:f=w674:string)
                    }
                  }
                }
              }
              "data" <- w386
              "字符串数值" <- w385
            }
            frame False {
            }
          }
          n284 = VISA Close(VISA resource name=w366, error in (no error)=w367) -> (error out=w364:errorcluster)
        }
        frame #2 {
          n285 = Tick Count (ms)() -> (millisecond timer value=w713:u32)
        }
        frame #3 {
          w735 = "\r\n"
          n286 = local read "命令"() -> (w731:string)
          n287 = local read "响应"() -> (w716:string)
          n288 = String To Byte Array(string=w731) -> (unsigned byte array=w732:u8[])
          n289 = case shown="\"假\", 默认" w715 {
            tunnel: [w740 w748 w749] -> w726
            tunnel: w716 -> [w739 w748 w749]
            frame "假", Default {
              n290 = String To Byte Array(string=w739) -> (unsigned byte array=w742:u8[])
              n291 = for {
                tunnel: w742 -> [w747] mode=indexing
                shift-right: [w745] -> w740
                shift-left: "" -> [w744]
                n292 = Number To Hexadecimal String(1:i16 2 ("宽度(-)"), 2:w747) -> (0:w746:string)
                n293 = Concatenate Strings(w744, w746) -> (w745:string)
              }
            }
            frame "启动自动化测试" {
            }
            frame "查询版本", "查询版本(长丰)" {
            }
          }
          n294 = for {
            tunnel: w732 -> [w758] mode=indexing
            shift-right: [w756] -> w730
            shift-left: "" -> [w755]
            n295 = Number To Hexadecimal String(1:i16 2 ("宽度(-)"), 2:w758) -> (0:w757:string)
            n296 = Concatenate Strings(w755, w757) -> (w756:string)
          }
          n297 = Unbundle By Name(w727) -> ("code"=w722:i32)
          n298 = Equal?(x=w722, y=-1073807253) -> (x = y?=w723:bool)
          n299 = Equal?(x=w722, y=-1073807298) -> (x = y?=w720:bool)
          n300 = Equal?(x=w722, y=-1073807252) -> (x = y?=w717:bool)
          n301 = Or(x=w723, y=w720) -> (x .or. y?=w718:bool)
          n302 = Or(x=w718, y=w717) -> (x .or. y?=w719:bool)
          n303 = case shown="假" w719 {
            tunnel: [w751 errorcluster {"status"=FALSE, "code"=0, "source"=""} ("t")] -> w728
            tunnel: w727 -> [w751 _]
            tunnel: w726 -> [w750 _]
            tunnel: [w750 ""] -> w725
            frame False {
            }
            frame True {
            }
          }
          n304 = Concatenate Strings("发送" ("字符串"), w715, ":" ("字符串"), w730, w735, "反馈:" ("字符串"), w725, w735) -> (→"CMD":string)
        }
        frame #4 {
          n305 = Tick Count (ms)() -> (millisecond timer value=w759:u32)
        }
      }
    }
  }
  "error out" <- w70
  n306 = Subtract(x=w66, y=w48) -> (x-y=→"x-y":u32)
